vi "SetValue.vi"(0 "reference in":refnum<class "AO.lvclass">, 5 "value":dbl format="%0.2f", 11 "error in (no error)":errorcluster) -> (4 "reference out":refnum<class "AO.lvclass">, 15 "error out":errorcluster)   [LabVIEW 2019, in "AO.lvclass"]
uses:
  AO.lvclass
  D:/GIT H4000/H4000/src/Proccess_class/Proccess.lvclass
  AO.lvclass/AO.ctl
  Proccess_class/Proccess.lvclass/Proccess.ctl
  Logger_class/Logger.lvclass/Logger.ctl
  Logger_class/Enqueue Signal.vi
  Proccess_class/GetNames.vi
  Proccess_class/GetLogger.vi
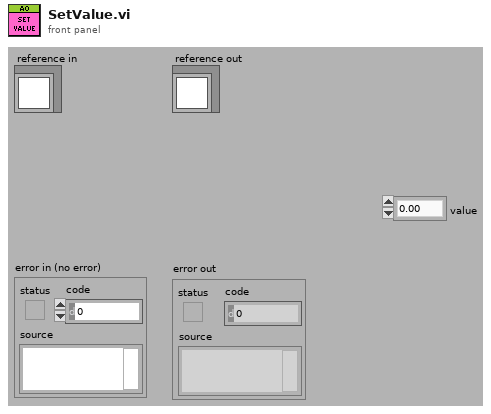
[diagram p1: front panel]
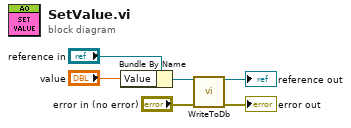
[diagram p0: block diagram]
diagram:
  n1 = Bundle By Name(cluster="reference in", "Value"="value") -> (w4:refnum<class "AO.lvclass">)
  n2 = call "WriteToDb.vi"("reference in"=w4, "error in (no error)"="error in (no error)") -> ("reference out"=→"reference out":refnum<class "AO.lvclass">, "error out"=→"error out":errorcluster)  [unwired: 12 in]
